vi "Get JSON Data.vi"(7 "Panel Origin":T1, 8 "error in (no error)":errorcluster, 9 "Force Get All Data":bool, 10 "VI Reference":refnum<vi>, 11 "Control In":refnum<class "Control.lvclass">) -> (0 "error out":errorcluster, 2 "JSON string":string, 3 "Control Out":refnum<class "Control.lvclass">)   [LabVIEW 2015, in "Front Panel Publisher.lvlib" / "Control.lvclass"]
uses:
  Control.lvclass
  <vilib>/Utility/miscctls.llb/LVPointTypeDef.ctl
  Object_class/Coordinates.ctl
  Object_class/Object.lvclass
  Front Panel Publisher.lvlib
  Web Front Panel_class/Web Front Panel.lvclass
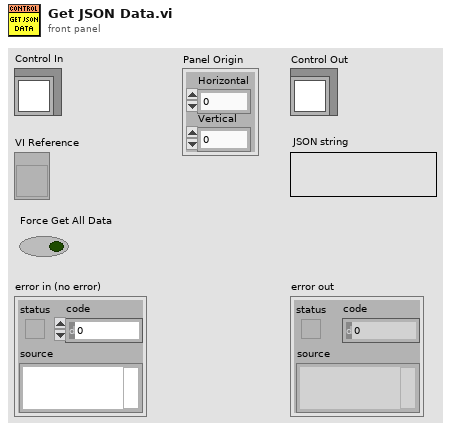
[diagram p1: front panel]
types:
  T1 = typedef "LVPointTypeDef.ctl" = cluster{"Horizontal":i16, "Vertical":i16}
  T2 = typedef "Front Panel Publisher.lvlib/Object.lvclass/Coordinates.ctl" = cluster{"Left":i32, "Top":i32, "Height":u32, "Width":u32}
  T3 = typedef "Front Panel Publisher.lvlib/Object.lvclass/Attributes.ctl" = cluster{"UID":i32, "Type":string, "Coordinates":T2, "Reference":refnum<vi>}
  T4 = typedef "LVRectTypeDef.ctl" = cluster{"Left":i16, "Top":i16, "Right":i16, "Bottom":i16}
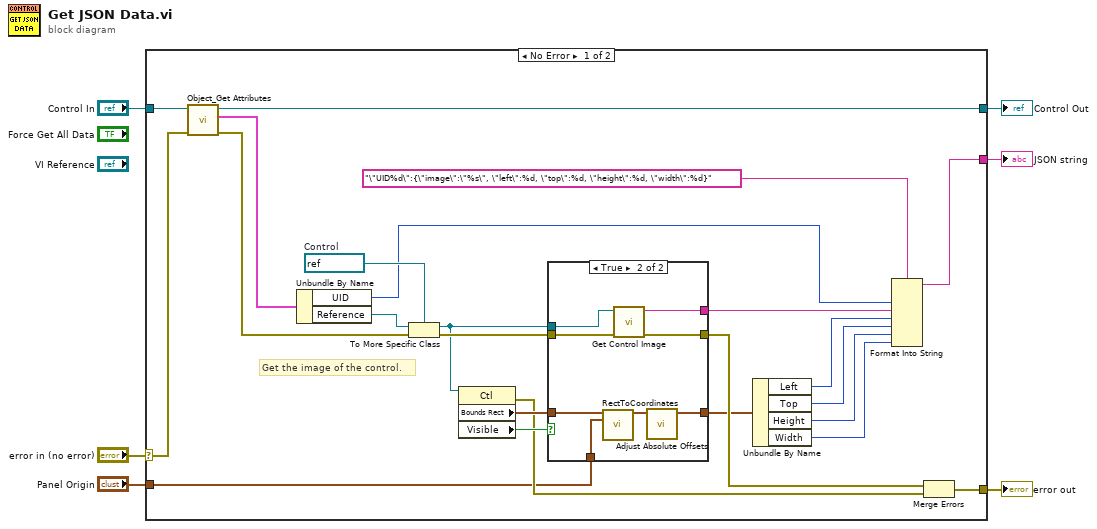
[diagram p0: block diagram]
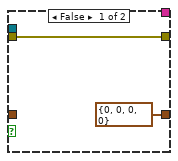
[diagram p2: hidden frame]
diagram:
  n1 = case shown="No Error" "error in (no error)" {
    selector: "error in (no error)" -> [w17 w42]
    tunnel: [w15 w42] -> w5
    tunnel: [w29 w41] -> w3
    tunnel: "Control In" -> [w16 w41]
    tunnel: [w25 _] -> w2
    tunnel: "Panel Origin" -> [w7 _]
    frame No Error {
      w27 = refnum<vi> refnum  # Control
      # "Get the image of the control."
      n2 = call "Object_Get Attributes.vi"("error in (no error)"=w17, "Object In"=w16) -> ("error out"=w23:errorcluster, "Data"=w30:T3, "Object Out"=w29:refnum<class "Control.lvclass">)  [unwired: 6 in, 1 out]
      n3 = Unbundle By Name(w30) -> ("UID"=w26:i32, "Reference"=w28:refnum<vi>)
      n4 = To More Specific Class(target class=w27, reference=w28, error in=w23) -> (specific class reference=w20:refnum<vi>, error out=w22:errorcluster)
      n5 = property class="Ctl"(reference=w20) -> (error out=w9:errorcluster, "Bounds Rect"=w21:T4, "Visible"=w18:bool)  [unwired: 1 in, 1 out]
      n6 = case shown="True" w18 {
        tunnel: [_ w40] -> w8
        tunnel: [w31 w39] -> w24
        tunnel: w22 -> [w31 w38]
        tunnel: w21 -> [_ w37]
        tunnel: w20 -> [_ w35]
        tunnel: [T2 {"Left"=0, "Top"=0, "Height"=0, "Width"=0} ("Coordinates out") w34] -> w19
        tunnel: w7 -> [_ w33]
        frame False {
        }
        frame True {
          n7 = call "RectToCoordinates.vi"("Rect"=w37, "Panel Origin"=w33) -> ("Coordinates"=w36:T2)  [unwired: 13 in]
          n8 = call "Get Control Image.vi"("error in (no error)"=w38, "Control ref"=w35) -> ("error out"=w39:errorcluster, "base64 encoded <img>"=w40:string)  [unwired: 7 in, 1 out]
          n9 = call "Adjust Absolute Offsets.vi"("Coordinates in"=w36) -> ("Coordinates out"=w34:T2)  [unwired: 8 in, 2 out]
        }
      }
      n10 = Unbundle By Name(w19) -> ("Left"=w13:i32, "Top"=w12:i32, "Height"=w11:u32, "Width"=w10:u32)
      n11 = Format Into String(format string="\"UID%d\":{\"image\":\"%s\", \"left\":%d, \"top\":%d, \"height\":%d, \"width\":%d}", w26, w8, w13, w12, w11, w10) -> (resulting string=w25:string)  [unwired: 2 in, 1 out]
      n12 = Merge Errors(w24, w9) -> (w15:errorcluster)
    }
    frame Error {
    }
  }
  "error out" <- w5
  "Control Out" <- w3
  "JSON string" <- w2
